vi "VRMSFreqAcqSubVI.vi"(8 "error in (no error)":errorcluster, 11 "Data Cluster in":T1) -> (0 "error out":errorcluster, 1 "freq":dbl format="%.2f", 2 "RMS value":dbl format="%0.2p", 3 "Data Cluster out":T1)   [LabVIEW 2017]
uses:
  Controls/ShiftRegisterCluster.ctl
  <vilib>/DAQmx/read.llb/DAQmx Read (Analog Wfm 1Chan NSamp).vi
  <vilib>/DAQmx/miscellaneous.llb/DAQmx Fill In Error Info.vi
  <vilib>/measure/madcrms.llb/Basic Averaged DC-RMS for 1 Chan.vi
  <vilib>/measure/NI_MAPro.lvlib
  <vilib>/gmath/NI_Gmath.lvlib
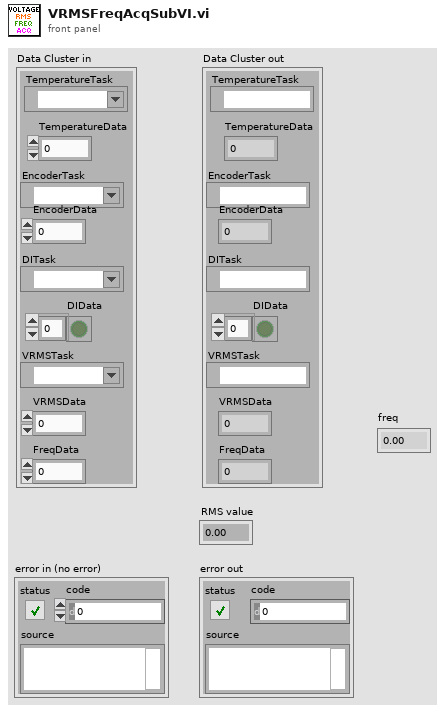
[diagram p1: front panel]
types:
  T1 = typedef "ShiftRegisterCluster.ctl" = cluster{"TemperatureTask":refnum<k21>, "TemperatureData":dbl, "EncoderTask":refnum<k21>, "EncoderData":dbl, "DITask":refnum<k21>, "DIData":bool[], "VRMSTask":refnum<k21>, "VRMSData":dbl, "FreqData":dbl}
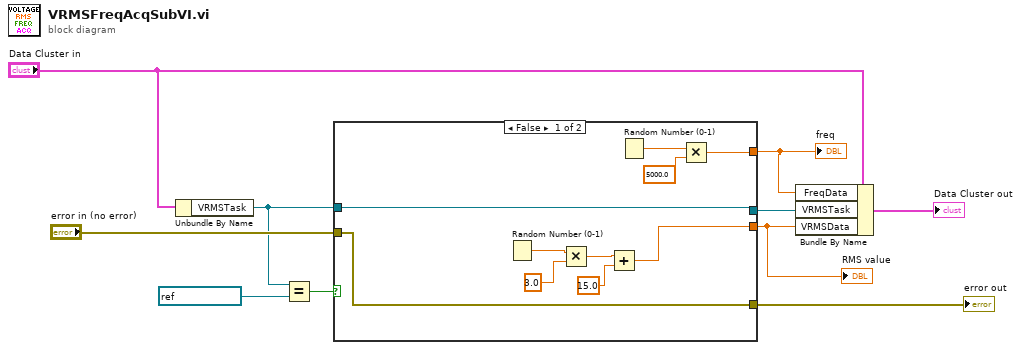
[diagram p0: block diagram]
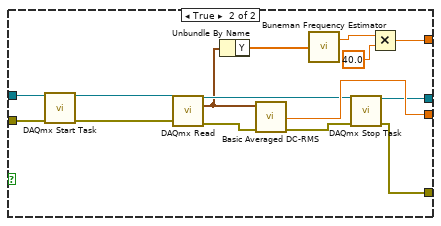
[diagram p2: hidden frame]
diagram:
  n1 = Unbundle By Name("Data Cluster in") -> ("VRMSTask"=w4:refnum<k21>)
  n2 = Equal?(x=w4, y=refnum<k21> "VRMSTask" ("DAQmx Task Name")) -> (x = y?=w2:bool)
  n3 = case shown="False" w2 {
    tunnel: [w15 w35] -> w10
    tunnel: [w20 w32] -> w8
    tunnel: [w14 w31] -> w6
    tunnel: "error in (no error)" -> [w14 w27]
    tunnel: w4 -> [w20 w26]
    tunnel: [w11 w21] -> w1
    frame False {
      n4 = Random Number (0-1)() -> (number: 0 to 1=w19:dbl)
      n5 = Multiply(x=w19, y=3.0) -> (x*y=w17:dbl)
      n6 = Add(x=w17, y=15.0) -> (x+y=w15:dbl)
      n7 = Random Number (0-1)() -> (number: 0 to 1=w13:dbl)
      n8 = Multiply(x=w13, y=5000.0) -> (x*y=w11:dbl)
    }
    frame True {
      n9 = call <vilib>:"DAQmx Start Task.vi"("task/channels in"=w26, "error in"=w27) -> ("task out"=w28:refnum<k21>, "error out"=w29:errorcluster)  [unwired: 12 in]
      n10 = call-poly <vilib>:"DAQmx Read.vi"("task/channels in"=w28, "error in"=w29) -> ("task out"=w30:refnum<k21>, "data"=w25:waveform(dbl), "error out"=w33:errorcluster)  [unwired: 11 in]
      n11 = Unbundle By Name(w25) -> ("Y"=w24:dbl[])
      n12 = call-poly <vilib>:"Basic Averaged DC-RMS.vi"("error in (no error)"=w33, "signal in"=w25) -> ("error out"=w34:errorcluster, "RMS value"=w35:dbl)  [unwired: 6 in, 2 out]
      n13 = call <vilib>:"Buneman Frequency Estimator.vi"("X"=w24) -> ("beta"=w23:dbl)  [unwired: 1 out]
      n14 = call <vilib>:"DAQmx Stop Task.vi"("task/channels in"=w30, "error in"=w34) -> ("task out"=w32:refnum<k21>, "error out"=w31:errorcluster)  [unwired: 12 in]
      n15 = Multiply(x=w23, y=40.0) -> (x*y=w21:dbl)
    }
  }
  "RMS value" <- w10
  "error out" <- w6
  "freq" <- w1
  n16 = Bundle By Name(cluster="Data Cluster in", "FreqData"=w1, "VRMSTask"=w8, "VRMSData"=w10) -> (→"Data Cluster out":T1)
